vi "Modbus to Cluster.vi"(1 "Modbus Req":T6, 2 "Output Data":dbl[](array[numeric]), 3 "Data Struct - All":T1) -> (0 "Data Struct - All Out":T1)   [LabVIEW 2020]
uses:
  Control/Data Struct - Display Data.ctl
  Control/Data Struct - SB.ctl
  Control/Data Struct - Bank.ctl
  Control/Data Struct - SI.ctl
  Control/Data Struct - PM.ctl
  Control/Device Name.ctl
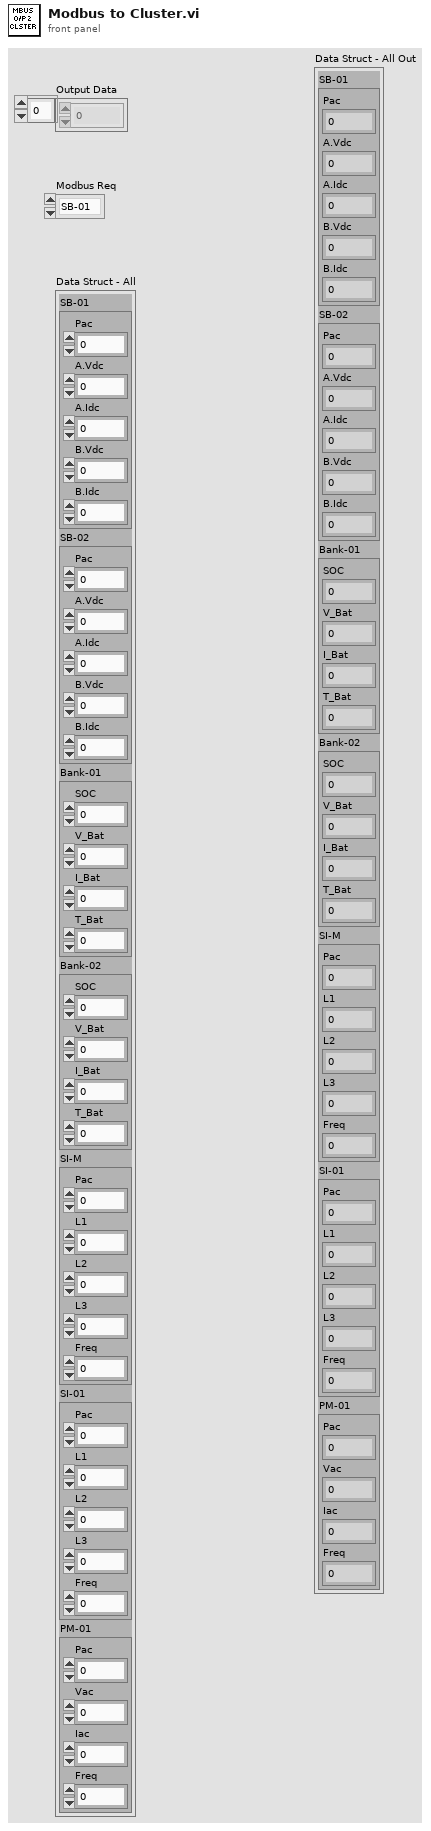
[diagram p1: front panel]
types:
  T1 = typedef "Data Struct - Display Data.ctl" = cluster{"SB-01":T2, "SB-02":T2, "Bank-01":T3, "Bank-02":T3, "SI-M":T4, "SI-01":T4, "PM-01":T5}
  T2 = typedef "Data Struct - SB.ctl" = cluster{"Pac":dbl, "A.Vdc":dbl, "A.Idc":dbl, "B.Vdc":dbl, "B.Idc":dbl}
  T3 = typedef "Data Struct - Bank.ctl" = cluster{"SOC":dbl, "V_Bat":dbl, "I_Bat":dbl, "T_Bat":dbl}
  T4 = typedef "Data Struct - SI.ctl" = cluster{"Pac":dbl, "L1":dbl, "L2":dbl, "L3":dbl, "Freq":dbl}
  T5 = typedef "Data Struct - PM.ctl" = cluster{"Pac":dbl, "Vac":dbl, "Iac":dbl, "Freq":dbl}
  T6 = typedef "Device Name.ctl" = enum16{"SB-01", "SB-02", "BANK-01", "BANK-02", "SI-M", "SI-01", "PM-01"}
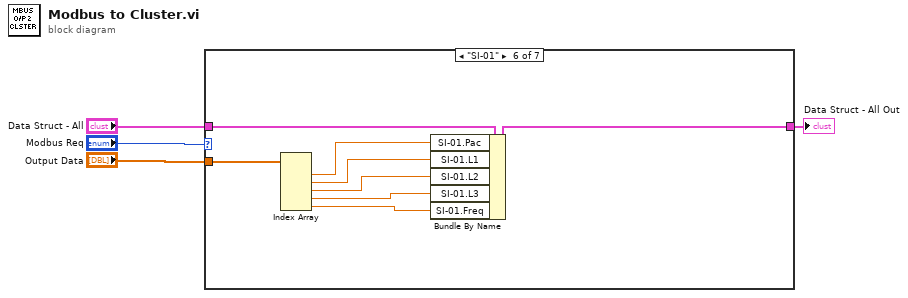
[diagram p0: block diagram]
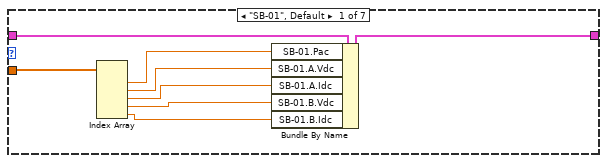
[diagram p2: hidden frame]
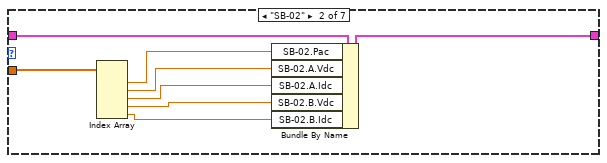
[diagram p3: hidden frame]
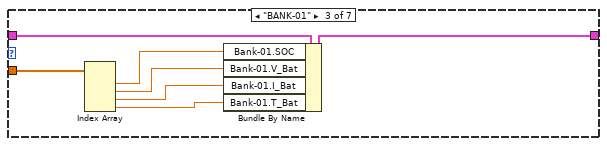
[diagram p4: hidden frame]
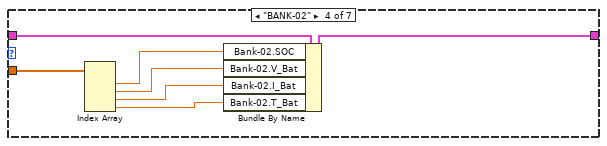
[diagram p5: hidden frame]
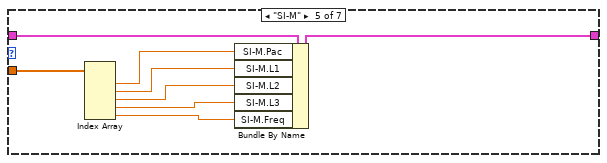
[diagram p6: hidden frame]
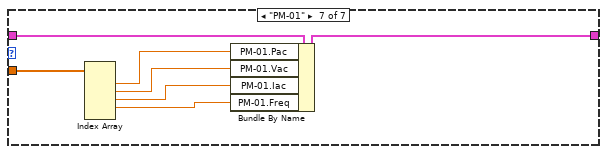
[diagram p7: hidden frame]
diagram:
  n1 = case shown="\"SI-01\"" "Modbus Req" {
    tunnel: "Output Data" -> [w10 w18 w26 w33 w41 w49 w56]
    tunnel: "Data Struct - All" -> [w12 w20 w27 w34 w42 w50 w57]
    tunnel: [w11 w19 w25 w32 w40 w48 w55] -> w1
    frame "SB-01", Default {
      n2 = Index Array(array=w10) -> (element #1=w9:dbl, element #2=w8:dbl, element #3=w7:dbl, element #4=w6:dbl, element #5=w5:dbl)  [unwired: 5 in]
      n3 = Bundle By Name(cluster=w12, "SB-01.Pac"=w9, "SB-01.A.Vdc"=w8, "SB-01.A.Idc"=w7, "SB-01.B.Vdc"=w6, "SB-01.B.Idc"=w5) -> (w11:T1)
    }
    frame "SB-02" {
      n4 = Index Array(array=w18) -> (element #1=w17:dbl, element #2=w16:dbl, element #3=w15:dbl, element #4=w14:dbl, element #5=w13:dbl)  [unwired: 5 in]
      n5 = Bundle By Name(cluster=w20, "SB-02.Pac"=w17, "SB-02.A.Vdc"=w16, "SB-02.A.Idc"=w15, "SB-02.B.Vdc"=w14, "SB-02.B.Idc"=w13) -> (w19:T1)
    }
    frame "BANK-01" {
      n6 = Index Array(array=w26) -> (element #1=w24:dbl, element #2=w23:dbl, element #3=w22:dbl, element #4=w21:dbl)  [unwired: 4 in]
      n7 = Bundle By Name(cluster=w27, "Bank-01.SOC"=w24, "Bank-01.V_Bat"=w23, "Bank-01.I_Bat"=w22, "Bank-01.T_Bat"=w21) -> (w25:T1)
    }
    frame "BANK-02" {
      n8 = Index Array(array=w33) -> (element #1=w31:dbl, element #2=w30:dbl, element #3=w29:dbl, element #4=w28:dbl)  [unwired: 4 in]
      n9 = Bundle By Name(cluster=w34, "Bank-02.SOC"=w31, "Bank-02.V_Bat"=w30, "Bank-02.I_Bat"=w29, "Bank-02.T_Bat"=w28) -> (w32:T1)
    }
    frame "SI-M" {
      n10 = Index Array(array=w41) -> (element #1=w39:dbl, element #2=w38:dbl, element #3=w37:dbl, element #4=w36:dbl, element #5=w35:dbl)  [unwired: 5 in]
      n11 = Bundle By Name(cluster=w42, "SI-M.Pac"=w39, "SI-M.L1"=w38, "SI-M.L2"=w37, "SI-M.L3"=w36, "SI-M.Freq"=w35) -> (w40:T1)
    }
    frame "SI-01" {
      n12 = Index Array(array=w49) -> (element #1=w47:dbl, element #2=w46:dbl, element #3=w45:dbl, element #4=w44:dbl, element #5=w43:dbl)  [unwired: 5 in]
      n13 = Bundle By Name(cluster=w50, "SI-01.Pac"=w47, "SI-01.L1"=w46, "SI-01.L2"=w45, "SI-01.L3"=w44, "SI-01.Freq"=w43) -> (w48:T1)
    }
    frame "PM-01" {
      n14 = Index Array(array=w56) -> (element #1=w54:dbl, element #2=w53:dbl, element #3=w52:dbl, element #4=w51:dbl)  [unwired: 5 in, 1 out]
      n15 = Bundle By Name(cluster=w57, "PM-01.Pac"=w54, "PM-01.Vac"=w53, "PM-01.Iac"=w52, "PM-01.Freq"=w51) -> (w55:T1)
    }
  }
  "Data Struct - All Out" <- w1
